vi "IR Test for MANU.vi"(0 "VISA resource name":refnum<visa-resource-name>, 5 "Configure RS232 Baud Rate":u32(ring)=115200 items=["9600"=9600, "19200"=19200, "38400"=38400, "57600"=57600, "115200"=115200], 7 "IR voltage(kV)":sgl=0.1 min=0.0499 max=1.0001 step=0.05 format="%.2f", 9 "Ramp Time":sgl=1.0 min=0.1 max=999.9 format="%.1f", 11 "IR Test Time(S)":sgl=1.0 min=1 max=999.9 format="%.1f", 12 "error in":errorcluster) -> (4 "VISA resource name out":refnum<visa-resource-name>, 6 "Voltage":string, 8 "Impedance":string, 10 "Time":string, 13 "Error Message":string, 14 "error out":errorcluster, 15 "PASS":bool)   [LabVIEW 2021, in "GPT-9000.lvlib"]
uses:
  <instrlib>/GPT-9800_GSB_L2011/GPT-9000.lvlib
panel:
  in  "IR reference value(M£[)":u16 max=9999
  in  "IR LO SET resistance value(M£[)":u16=2 min=1 max=9999
  in  "IR HI SET resistance value(M£[)":u16=9999 min=2 max=9999
  in  "Sets value to high impedance":u8(ring) items=["High Impedance"=1, "Setup as below"=0]
  in  "Clear Error(True)":bool=TRUE
  in  "ID Query (True)":bool=TRUE
  out "ID Return String":string
  in  "Start":bool
  in  "Stop":bool
  in  "Test number":u8 max=100
  out "Error LED":bool
  in  "Test name":string="TEST_NAME"
  out "READY":bool
  out "TEST":bool
  out "FAIL":bool
  out "LED":bool
  out "Ready to Start":bool
  # "IR Test for MANU Mode"
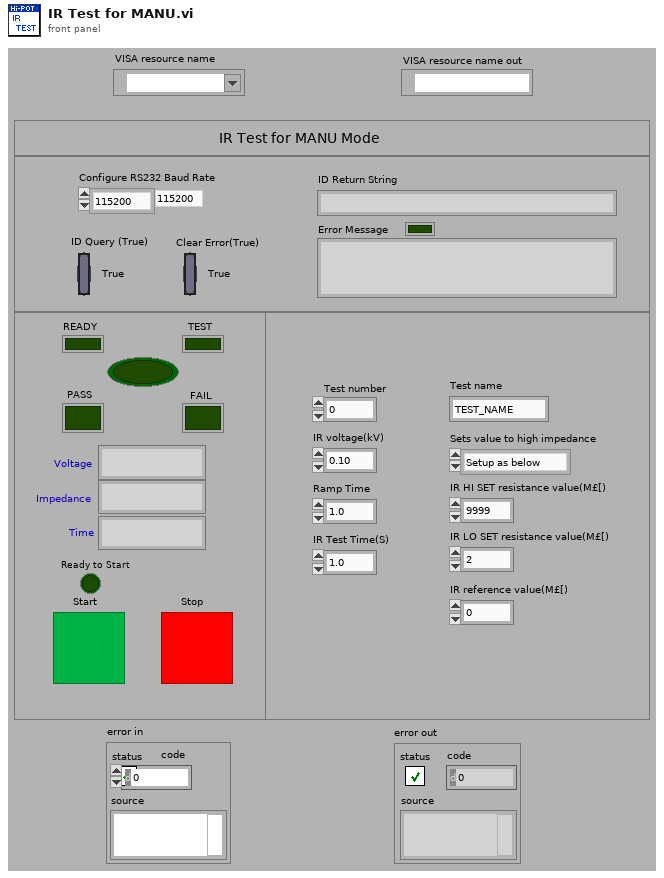
[diagram p1: front panel]
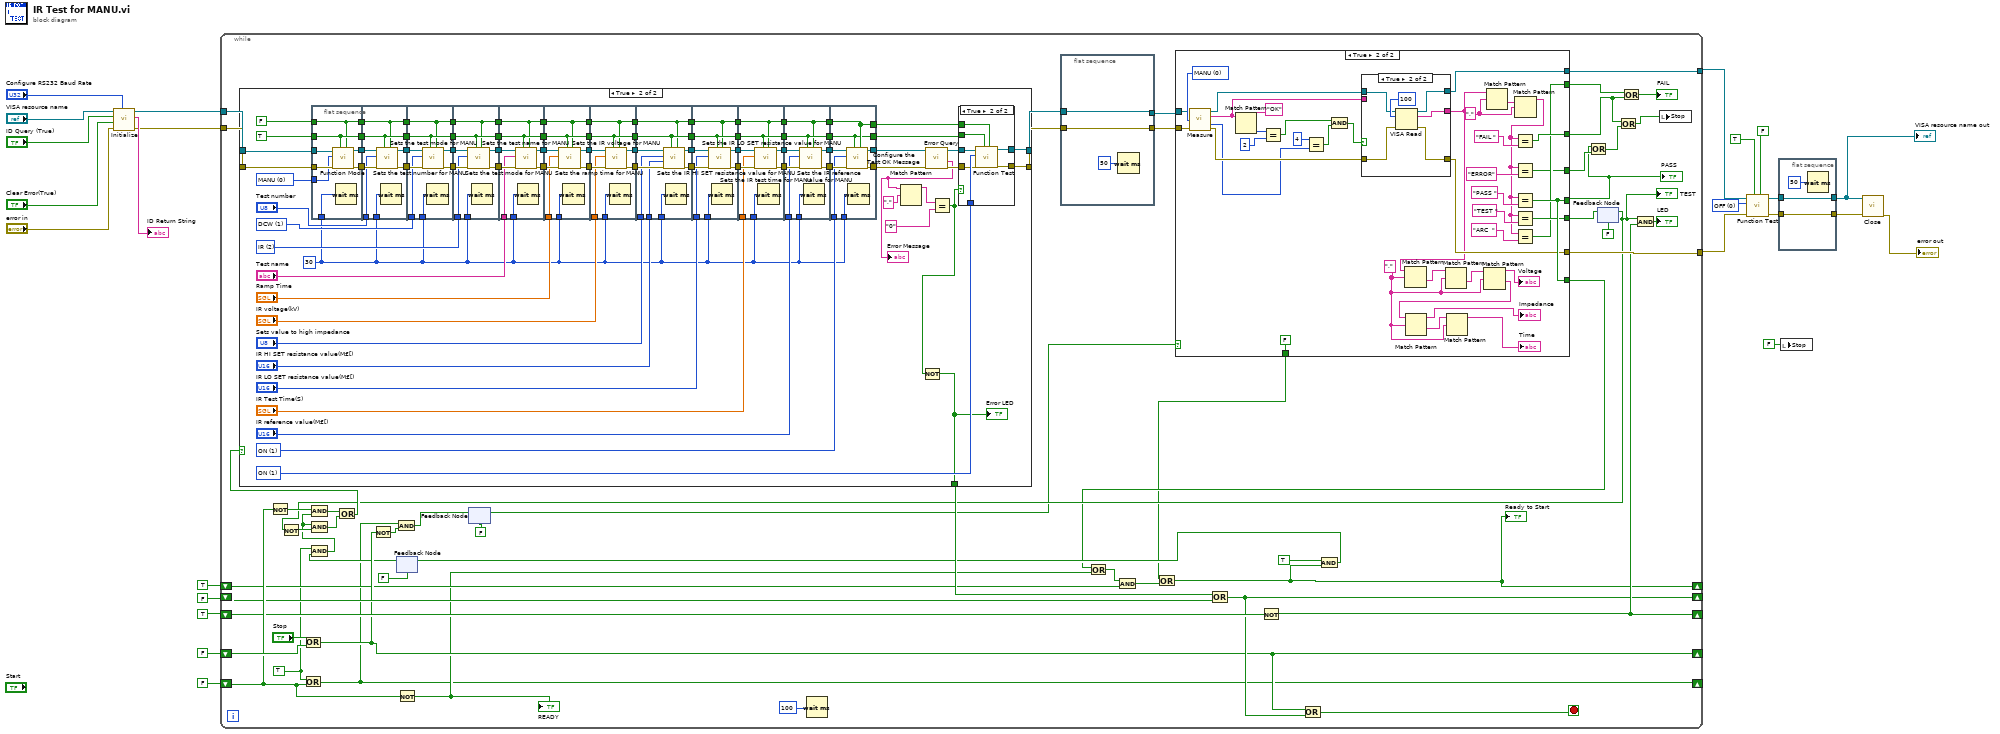
[diagram p0: block diagram]
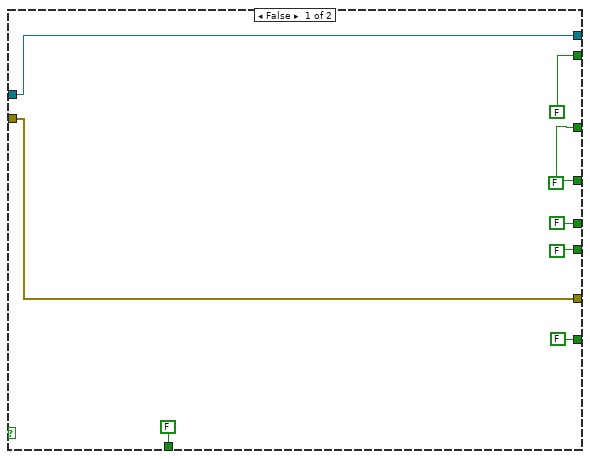
[diagram p2: hidden frame]
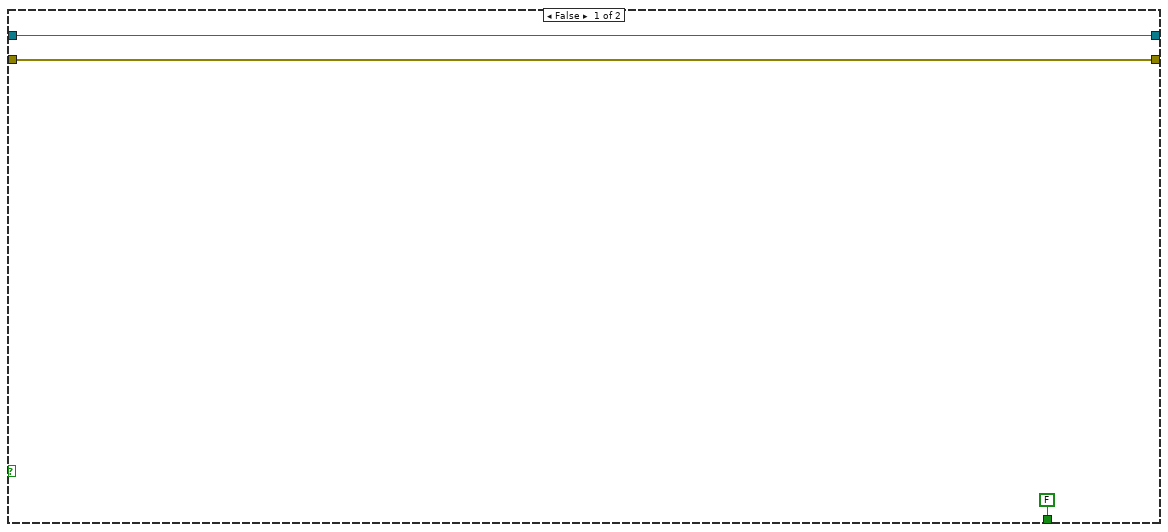
[diagram p4: hidden frame]
diagram:
  w22 = u8 0 items=["OFF", "ON"] ("Function Test")
  n1 = call <instrlib>:"Initialize.vi"("Configure RS232 Baud Rate"="Configure RS232 Baud Rate", "error in (no error)"="error in", "Clear Error(True)"="Clear Error(True)", "ID Query (True)"="ID Query (True)", "VISA resource name"="VISA resource name") -> ("error out"=w11:errorcluster, "ID Return String"=→"ID Return String":string, "VISA resource name out"=w12:refnum<visa-resource-name>)  [unwired: 3 in, 1 out]
  n2 = while {
    shift-right: [w39] -> _
    shift-left: FALSE -> [w70]
    shift-right: [w55] -> _
    shift-left: FALSE -> [w76]
    tunnel: [w75] -> w24
    tunnel: [w74] -> w23
    shift-right: [w69] -> _
    shift-left: TRUE -> [w68]
    tunnel: w12 -> [w62]
    tunnel: w11 -> [w61]
    shift-right: [w58] -> _
    shift-left: FALSE -> [w59]
    shift-right: [w46] -> _
    shift-left: TRUE -> [w50]
    stop <- w60 stop-if-true
    w32 = TRUE ("x")
    n3 = Not(x=w70) -> (.not. x?=w73:bool)
    n4 = Or(x="Stop", y=w76) -> (x .or. y?=w55:bool)
    n5 = Or(x=w32, y=w70) -> (x .or. y?=w39:bool)
    n6 = Not(x=w55) -> (.not. x?=w72:bool)
    n7 = And(x=w39, y=w72) -> (x .and. y?=w71:bool)
    n8 = feedback #1(FALSE) -> (w44:bool)
    n9 = And(x=w32, y=w44) -> (x .and. y?=w47:bool)
    n10 = And(x=w73, y=w47) -> (x .and. y?=w65:bool)
    n11 = Not(x=w70) -> (.not. x?=w48:bool)
    "READY" <- w48
    n12 = feedback-in #2(w71) -> ()
    n13 = feedback #2(FALSE) -> (w38:bool)
    n14 = Wait (ms)(milliseconds to wait=u32 100) -> ()  [unwired: 1 out]
    n15 = flat-sequence {
      tunnel: w36 -> [w80]
      tunnel: [w80] -> w35
      tunnel: w34 -> [w79]
      tunnel: [w79] -> w33
      frame #0 {
        n16 = Wait (ms)(milliseconds to wait=u32 50) -> ()  [unwired: 1 out]
      }
    }
    n17 = case shown="True" w38 {
      tunnel: [w83 w96] -> w75
      tunnel: [w82 w95] -> w74
      tunnel: [FALSE w113] -> w41
      tunnel: [w81 w122] -> w28
      tunnel: [FALSE w113] -> w26
      tunnel: [FALSE w112] -> w54
      tunnel: [FALSE w110] -> w29
      tunnel: w35 -> [w83 w98]
      tunnel: w33 -> [w82 w97]
      tunnel: [FALSE FALSE] -> w37
      tunnel: [w81 w89] -> w27
      frame False {
        w81 = FALSE
      }
      frame True {
        w109 = u8 0 items=["MANU", "AUTO"] ("Function Mode Numeric")
        w114 = "," ("regular expression")
        w124 = "," ("regular expression")
        n18 = call <instrlib>:"Measure.vi"("VISA resource name"=w98, "Function Mode Numeric"=w109, "error in"=w97) -> ("VISA resource name out"=w105:refnum<visa-resource-name>, "Return  the test status"=w99:string, "Return the String Count"=w101:u16, "error out"=w104:errorcluster)  [unwired: 9 in]
        n19 = Match Pattern(string=w99, regular expression="OK") -> (offset past match=w107:i32)  [unwired: 1 in, 3 out]
        n20 = Equal?(x=w107, y=2) -> (x = y?=w93:bool)
        n21 = Equal?(x=u16 4, y=w101) -> (x = y?=w102:bool)
        n22 = And(x=w93, y=w102) -> (x .and. y?=w103:bool)
        n23 = case shown="True" w103 {
          tunnel: w104 -> [w130 w131]
          tunnel: [w129 w135] -> w96
          tunnel: [w130 w134] -> w95
          tunnel: [w128 w133] -> w94
          tunnel: w105 -> [w129 w132]
          tunnel: w99 -> [w128 _]
          frame False {
          }
          frame True {
            n24 = VISA Read(VISA resource name=w132, byte count=u32 100, error in (no error)=w131) -> (VISA resource name out=w135:refnum<visa-resource-name>, read buffer=w133:string, error out=w134:errorcluster)  [unwired: 1 out]
          }
        }
        n25 = Match Pattern(string=w94, regular expression=w114) -> (after substring=w121:string)  [unwired: 1 in, 3 out]
        n26 = Match Pattern(string=w121, regular expression=w114) -> (after substring=w117:string)  [unwired: 1 in, 3 out]
        n27 = Match Pattern(string=w117, regular expression=w114) -> (before substring=→"Voltage":string, after substring=w115:string)  [unwired: 1 in, 2 out]
        n28 = Match Pattern(string=w115, regular expression=w114) -> (before substring=→"Impedance":string, after substring=w120:string)  [unwired: 1 in, 2 out]
        n29 = Match Pattern(string=w120, regular expression=w114) -> (before substring=→"Time":string)  [unwired: 1 in, 3 out]
        n30 = Match Pattern(string=w94, regular expression=w124) -> (after substring=w125:string)  [unwired: 1 in, 3 out]
        n31 = Match Pattern(string=w125, regular expression=w124) -> (before substring=w90:string)  [unwired: 1 in, 3 out]
        n32 = Equal?(x=w90, y="FAIL ") -> (x = y?=w122:bool)
        n33 = Equal?(x=w90, y="ERROR") -> (x = y?=w89:bool)
        n34 = Equal?(x=w90, y="PASS ") -> (x = y?=w113:bool)
        n35 = Equal?(x=w90, y="TEST ") -> (x = y?=w112:bool)
        n36 = Equal?(x=w90, y="ARC  ") -> (x = y?=w110:bool)
      }
    }
    "PASS" <- w26
    n37 = Or(x=w41, y=w48) -> (x .or. y?=w49:bool)
    n38 = And(x=w49, y=w50) -> (x .and. y?=w51:bool)
    n39 = Or(x=w37, y=w51) -> (x .or. y?=w46:bool)
    "Ready to Start" <- w46
    n40 = Not(x=w68) -> (.not. x?=w69:bool)
    n41 = And(x=TRUE, y=w46) -> (x .and. y?=w42:bool)
    n42 = feedback-in #1(w42) -> ()
    n43 = Or(x=w26, y=w27) -> (x .or. y?=w25:bool)
    n44 = feedback-in #3(w54) -> ()
    n45 = feedback #3(FALSE) -> (w53:bool)
    "TEST" <- w53
    n46 = Not(x=w53) -> (.not. x?=w63:bool)
    n47 = And(x=w47, y=w63) -> (x .and. y?=w64:bool)
    n48 = Or(x=w65, y=w64) -> (x .or. y?=w56:bool)
    n49 = case shown="True" w56 {
      tunnel: w62 -> [w139 w205]
      tunnel: w61 -> [w138 w204]
      tunnel: [w139 w213] -> w36
      tunnel: [w138 w212] -> w34
      tunnel: [FALSE w206] -> w57
      frame False {
      }
      frame True {
        w140 = u32 30 ("milliseconds to wait")
        w151 = u8 1 items=["ACW", "DCW", "IR", "GB"] ("Test Mode")
        w141 = u8 1 items=["OFF", "ON"] ("Send Message when test stop")
        w150 = u8 2 items=["ACW", "DCW", "IR", "GB"] ("Test Mode")
        w153 = u8 0 items=["AUTO"=1, "MANU"=0] ("Function Mode")
        w216 = u8 1 items=["OFF", "ON"] ("Function Test")
        n50 = flat-sequence {
          tunnel: w205 -> [w224]
          tunnel: w204 -> [w223]
          tunnel: [w222] -> w203
          tunnel: [w221] -> w202
          tunnel: TRUE -> [w220]
          tunnel: FALSE -> [w219]
          tunnel: [w220] -> w167
          tunnel: [w219] -> w156
          tunnel: w153 -> [w218]
          tunnel: w140 -> [w217]
          tunnel: w203 -> [w232]
          tunnel: w202 -> [w231]
          tunnel: [w230] -> w201
          tunnel: [w229] -> w200
          tunnel: [w228] -> w168
          tunnel: w167 -> [w228]
          tunnel: [w227] -> w157
          tunnel: w156 -> [w227]
          tunnel: "Test number" -> [w226]
          tunnel: w140 -> [w225]
          tunnel: w201 -> [w240]
          tunnel: w200 -> [w239]
          tunnel: [w238] -> w199
          tunnel: [w237] -> w198
          tunnel: [w236] -> w169
          tunnel: w168 -> [w236]
          tunnel: [w235] -> w158
          tunnel: w157 -> [w235]
          tunnel: w151 -> [w234]
          tunnel: w140 -> [w233]
          tunnel: w199 -> [w248]
          tunnel: w198 -> [w247]
          tunnel: [w246] -> w197
          tunnel: [w245] -> w196
          tunnel: [w244] -> w170
          tunnel: w169 -> [w244]
          tunnel: [w243] -> w159
          tunnel: w158 -> [w243]
          tunnel: w150 -> [w242]
          tunnel: w140 -> [w241]
          tunnel: w197 -> [w256]
          tunnel: w196 -> [w255]
          tunnel: [w254] -> w195
          tunnel: [w253] -> w194
          tunnel: [w252] -> w171
          tunnel: w170 -> [w252]
          tunnel: [w251] -> w160
          tunnel: w159 -> [w251]
          tunnel: "Test name" -> [w250]
          tunnel: w140 -> [w249]
          tunnel: w195 -> [w264]
          tunnel: w194 -> [w263]
          tunnel: [w262] -> w193
          tunnel: [w261] -> w192
          tunnel: [w260] -> w172
          tunnel: w171 -> [w260]
          tunnel: [w259] -> w161
          tunnel: w160 -> [w259]
          tunnel: "Ramp Time" -> [w258]
          tunnel: w140 -> [w257]
          tunnel: w193 -> [w272]
          tunnel: w192 -> [w271]
          tunnel: [w270] -> w191
          tunnel: [w269] -> w190
          tunnel: [w268] -> w173
          tunnel: w172 -> [w268]
          tunnel: [w267] -> w162
          tunnel: w161 -> [w267]
          tunnel: "IR voltage(kV)" -> [w266]
          tunnel: w140 -> [w265]
          tunnel: w191 -> [w281]
          tunnel: w190 -> [w280]
          tunnel: [w279] -> w189
          tunnel: [w278] -> w188
          tunnel: [w277] -> w174
          tunnel: w173 -> [w277]
          tunnel: [w276] -> w163
          tunnel: w162 -> [w276]
          tunnel: "Sets value to high impedance" -> [w275]
          tunnel: "IR HI SET resistance value(M£[)" -> [w274]
          tunnel: w140 -> [w273]
          tunnel: w189 -> [w289]
          tunnel: w188 -> [w288]
          tunnel: [w287] -> w187
          tunnel: [w286] -> w186
          tunnel: [w285] -> w175
          tunnel: w174 -> [w285]
          tunnel: [w284] -> w164
          tunnel: w163 -> [w284]
          tunnel: "IR LO SET resistance value(M£[)" -> [w283]
          tunnel: w140 -> [w282]
          tunnel: w187 -> [w297]
          tunnel: w186 -> [w296]
          tunnel: [w295] -> w185
          tunnel: [w294] -> w184
          tunnel: [w293] -> w176
          tunnel: w175 -> [w293]
          tunnel: [w292] -> w165
          tunnel: w164 -> [w292]
          tunnel: "IR Test Time(S)" -> [w291]
          tunnel: w140 -> [w290]
          tunnel: w185 -> [w305]
          tunnel: w184 -> [w304]
          tunnel: [w303] -> w183
          tunnel: [w302] -> w182
          tunnel: [w301] -> w177
          tunnel: w176 -> [w301]
          tunnel: [w300] -> w166
          tunnel: w165 -> [w300]
          tunnel: "IR reference value(M£[)" -> [w299]
          tunnel: w140 -> [w298]
          tunnel: w183 -> [w313]
          tunnel: w182 -> [w312]
          tunnel: [w311] -> w181
          tunnel: [w310] -> w180
          tunnel: w177 -> [w308]
          tunnel: w166 -> [w309]
          tunnel: [w309] -> w155
          tunnel: [w308] -> w154
          tunnel: w141 -> [w307]
          tunnel: w140 -> [w306]
          frame #0 {
            n51 = call <instrlib>:"Function Mode.vi"("Enable to Query"=w219, "Enable to Setup"=w220, "error in"=w223, "Function Mode"=w218, "VISA resource name"=w224) -> ("error out"=w221:errorcluster, "VISA resource name out"=w222:refnum<visa-resource-name>)  [unwired: 4 in, 1 out]
            n52 = Wait (ms)(milliseconds to wait=w217) -> ()  [unwired: 1 out]
          }
          frame #1 {
            n53 = call <instrlib>:"Sets the test number for MANU.vi"("Enable to Query"=w227, "Enable to Setup"=w228, "error in"=w231, "Test number"=w226, "VISA resource name"=w232) -> ("error out"=w229:errorcluster, "VISA resource name out"=w230:refnum<visa-resource-name>)  [unwired: 4 in, 1 out]
            n54 = Wait (ms)(milliseconds to wait=w225) -> ()  [unwired: 1 out]
          }
          frame #2 {
            n55 = call <instrlib>:"Sets the test mode for MANU.vi"("Enable to Query"=w235, "Enable to Setup"=w236, "error in"=w239, "Test Mode"=w234, "VISA resource name"=w240) -> ("error out"=w237:errorcluster, "VISA resource name out"=w238:refnum<visa-resource-name>)  [unwired: 4 in, 1 out]
            n56 = Wait (ms)(milliseconds to wait=w233) -> ()  [unwired: 1 out]
          }
          frame #3 {
            n57 = call <instrlib>:"Sets the test mode for MANU.vi"("Enable to Query"=w243, "Enable to Setup"=w244, "error in"=w247, "Test Mode"=w242, "VISA resource name"=w248) -> ("error out"=w245:errorcluster, "VISA resource name out"=w246:refnum<visa-resource-name>)  [unwired: 4 in, 1 out]
            n58 = Wait (ms)(milliseconds to wait=w241) -> ()  [unwired: 1 out]
          }
          frame #4 {
            n59 = call <instrlib>:"Sets the test name for MANU.vi"("Enable to Query"=w251, "Enable to Setup"=w252, "error in"=w255, "Test name"=w250, "VISA resource name"=w256) -> ("error out"=w253:errorcluster, "VISA resource name out"=w254:refnum<visa-resource-name>)  [unwired: 4 in, 1 out]
            n60 = Wait (ms)(milliseconds to wait=w249) -> ()  [unwired: 1 out]
          }
          frame #5 {
            n61 = call <instrlib>:"Sets the ramp time for MANU.vi"("Enable to Query"=w259, "Enable to Setup"=w260, "error in"=w263, "Ramp Time"=w258, "VISA resource name"=w264) -> ("error out"=w261:errorcluster, "VISA resource name out"=w262:refnum<visa-resource-name>)  [unwired: 4 in, 1 out]
            n62 = Wait (ms)(milliseconds to wait=w257) -> ()  [unwired: 1 out]
          }
          frame #6 {
            n63 = call <instrlib>:"Sets the IR voltage for MANU.vi"("Enable to Query"=w267, "Enable to Setup"=w268, "error in"=w271, "IR voltage(kV)"=w266, "VISA resource name"=w272) -> ("error out"=w269:errorcluster, "VISA resource name out"=w270:refnum<visa-resource-name>)  [unwired: 4 in, 1 out]
            n64 = Wait (ms)(milliseconds to wait=w265) -> ()  [unwired: 1 out]
          }
          frame #7 {
            n65 = call <instrlib>:"Sets the IR HI SET resistance value for MANU.vi"("Enable to Query"=w276, "Enable to Setup"=w277, "error in"=w280, "IR HI SET resistance value(M£[)"=w274, "Sets value to high impedance"=w275, "VISA resource name"=w281) -> ("error out"=w278:errorcluster, "VISA resource name out"=w279:refnum<visa-resource-name>)  [unwired: 3 in, 1 out]
            n66 = Wait (ms)(milliseconds to wait=w273) -> ()  [unwired: 1 out]
          }
          frame #8 {
            n67 = call <instrlib>:"Sets the IR LO SET resistance value for MANU.vi"("Enable to Query"=w284, "Enable to Setup"=w285, "error in"=w288, "IR LO SET resistance value(M£[)"=w283, "VISA resource name"=w289) -> ("error out"=w286:errorcluster, "VISA resource name out"=w287:refnum<visa-resource-name>)  [unwired: 4 in, 1 out]
            n68 = Wait (ms)(milliseconds to wait=w282) -> ()  [unwired: 1 out]
          }
          frame #9 {
            n69 = call <instrlib>:"Sets the IR test time for MANU.vi"("Enable to Query"=w292, "Enable to Setup"=w293, "error in"=w296, "IR Test Time(S)"=w291, "VISA resource name"=w297) -> ("error out"=w294:errorcluster, "VISA resource name out"=w295:refnum<visa-resource-name>)  [unwired: 4 in, 1 out]
            n70 = Wait (ms)(milliseconds to wait=w290) -> ()  [unwired: 1 out]
          }
          frame #10 {
            n71 = call <instrlib>:"Sets the IR reference value for MANU.vi"("Enable to Query"=w300, "Enable to Setup"=w301, "error in"=w304, "IR reference value(M£[)"=w299, "VISA resource name"=w305) -> ("error out"=w302:errorcluster, "VISA resource name out"=w303:refnum<visa-resource-name>)  [unwired: 4 in, 1 out]
            n72 = Wait (ms)(milliseconds to wait=w298) -> ()  [unwired: 1 out]
          }
          frame #11 {
            n73 = call <instrlib>:"Configure the Test OK Message.vi"("Query the Message"=w309, "Setup the Message"=w308, "error in"=w312, "Send Message when test stop"=w307, "VISA resource name"=w313) -> ("error out"=w310:errorcluster, "VISA resource name out"=w311:refnum<visa-resource-name>)  [unwired: 4 in, 1 out]
            n74 = Wait (ms)(milliseconds to wait=w306) -> ()  [unwired: 1 out]
          }
        }
        n75 = call <instrlib>:"Error Query.vi"("error in (no error)"=w180, "VISA resource name"=w181) -> ("error out"=w214:errorcluster, "Error Message"=w208:string, "VISA resource name out"=w215:refnum<visa-resource-name>)  [unwired: 6 in, 1 out]
        "Error Message" <- w208
        n76 = Match Pattern(string=w208, regular expression=",") -> (before substring=w210:string)  [unwired: 1 in, 3 out]
        n77 = Equal?(x=w210, y="0") -> (x = y?=w207:bool)
        n78 = Not(x=w207) -> (.not. x?=w206:bool)
        "Error LED" <- w206
        n79 = case shown="True" w207 {
          tunnel: w216 -> [_ w322]
          tunnel: w215 -> [w315 w321]
          tunnel: w214 -> [w314 w320]
          tunnel: [w315 w319] -> w213
          tunnel: [w314 w318] -> w212
          tunnel: w154 -> [_ w317]
          tunnel: w155 -> [_ w316]
          frame False {
          }
          frame True {
            n80 = call <instrlib>:"Function Test.vi"("VISA resource name"=w321, "Function Test"=w322, "error in"=w320, "Enable to Setup"=w317, "Enable to Query"=w316) -> ("VISA resource name out"=w319:refnum<visa-resource-name>, "error out"=w318:errorcluster)  [unwired: 3 in, 1 out]
          }
        }
      }
    }
    n81 = Or(x=w57, y=w59) -> (x .or. y?=w58:bool)
    n82 = Or(x=w55, y=w58) -> (x .or. y?=w60:bool)
    n83 = Or(x=w28, y=w25) -> (x .or. y?=w31:bool)
    n84 = Or(x=w29, y=w28) -> (x .or. y?=→"FAIL":bool)
    n85 = And(x=w53, y=w69) -> (x .and. y?=→"LED":bool)
    n86 = local write "Stop"(w31) -> ()
  }
  n87 = call <instrlib>:"Function Test.vi"("VISA resource name"=w24, "Function Test"=w22, "error in"=w23, "Enable to Setup"=TRUE, "Enable to Query"=FALSE) -> ("VISA resource name out"=w6:refnum<visa-resource-name>, "error out"=w4:errorcluster)  [unwired: 3 in, 1 out]
  n88 = flat-sequence {
    tunnel: w6 -> [w325]
    tunnel: [w325] -> w5
    tunnel: w4 -> [w324]
    tunnel: [w324] -> w3
    frame #0 {
      n89 = Wait (ms)(milliseconds to wait=u32 50) -> ()  [unwired: 1 out]
    }
  }
  n90 = local write "Stop"(FALSE ("Stop")) -> ()
  n91 = call <instrlib>:"Close.vi"("error in (no error)"=w3, "VISA resource name"=w5) -> ("error out"=→"error out":errorcluster)  [unwired: 9 in]
  "VISA resource name out" <- w5
